vi "Read Combination.vi"(8 "error in (no error)":errorcluster, 11 "Cheat in":refnum<class "Cheat.lvclass">) -> (0 "error out":errorcluster, 2 "Combination":T1[](array[typedef]), 3 "Cheat out":refnum<class "Cheat.lvclass">)   [LabVIEW 2019, in "RT_Game.lvlib" / "Cheat.lvclass"]
uses:
  Cheat.lvclass
  CheatControl.ctl
  Cheat.lvclass/Cheat.ctl
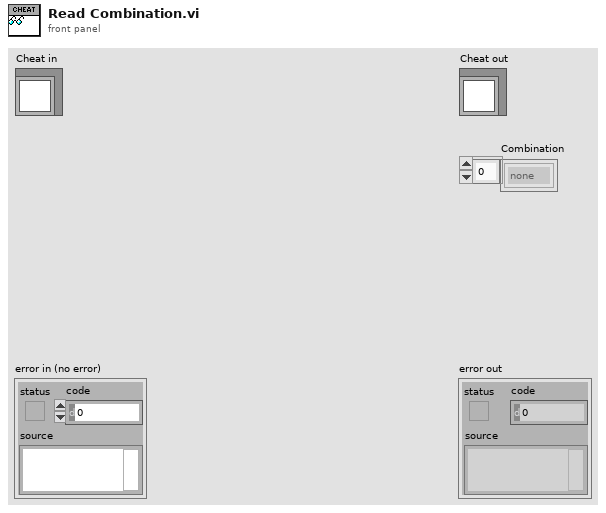
[diagram p1: front panel]
types:
  T1 = typedef "RT_Game.lvlib/Cheat.lvclass/CheatControl.ctl" = enum16{"none", "left1", "left2", "right1", "right2", "leftStick", "rightStick"}
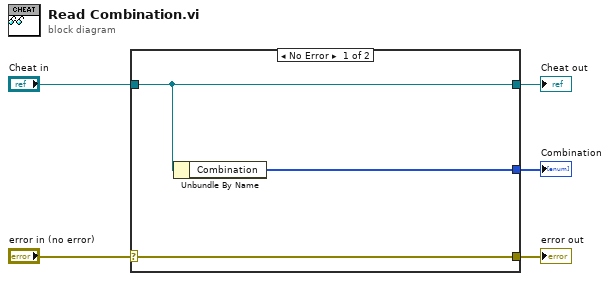
[diagram p0: block diagram]
diagram:
  n1 = case shown="No Error" "error in (no error)" {
    selector: "error in (no error)" -> [w8 w9]
    tunnel: [w8 w9] -> w4
    tunnel: [w7 w10] -> w2
    tunnel: "Cheat in" -> [w7 w10]
    tunnel: [w6 _] -> w1
    frame No Error {
      n2 = Unbundle By Name(w7) -> ("Combination"=w6:T1[])
    }
    frame Error {
    }
  }
  "error out" <- w4
  "Cheat out" <- w2
  "Combination" <- w1
